vi "testing_waveforms.vi"() -> ()   [LabVIEW 2019, in "mmW_commands.lvlib"]
uses:
  mmW_commands.lvlib
  <vilib>/measure/maspectr.llb/FFT Power Spectrum and PSD for 1 Chan.vi
  <vilib>/measure/NI_MAPro.lvlib
  <vilib>/Analysis/NI_AALBase.lvlib
panel:
  out "theta":dbl[](graph)
  out "r":dbl[](graph)
  in  "cycles":dbl(slide)=400.0 scale=0.0..400.0
  out "Power Spectrum / PSD":cluster{"f0":dbl, "df":dbl, "magnitude":dbl[]}(graph)
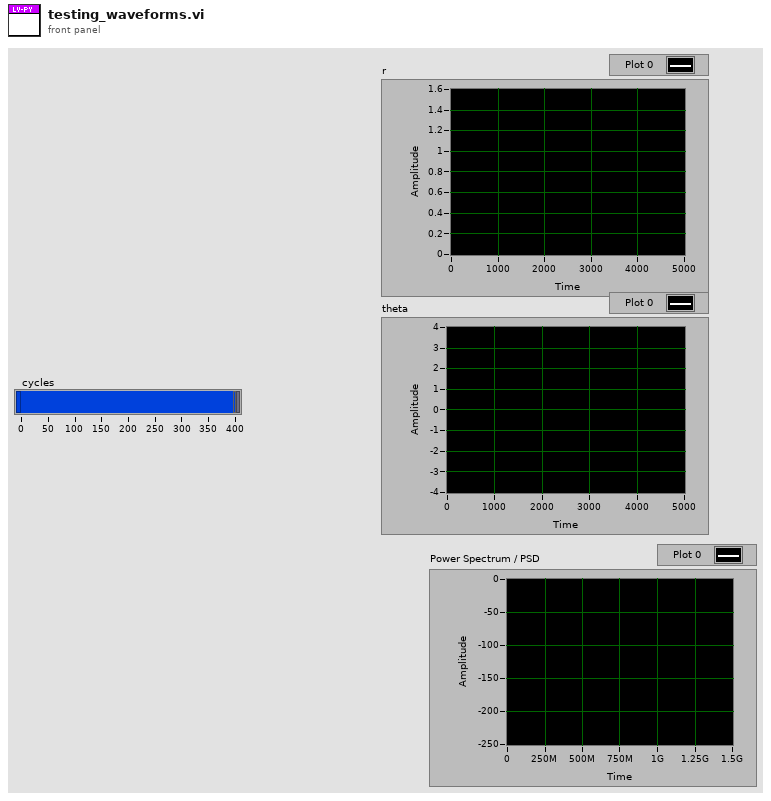
[diagram p1: front panel]
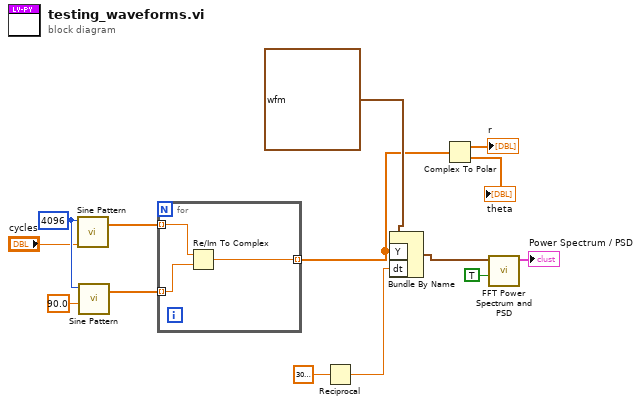
[diagram p0: block diagram]
diagram:
  w13 = 4096 ("samples")
  n1 = call <vilib>:"Sine Pattern.vi"("cycles"="cycles", "samples"=w13) -> ("Sinusoidal Pattern"=w12:dbl[])  [unwired: 2 in, 1 out]
  n2 = call <vilib>:"Sine Pattern.vi"("phase(degrees)"=90.0, "samples"=w13) -> ("Sinusoidal Pattern"=w11:dbl[])  [unwired: 2 in, 1 out]
  n3 = for {
    tunnel: w12 -> [w17] mode=indexing
    tunnel: w11 -> [w16] mode=indexing
    tunnel: [w15] -> w3 mode=indexing
    n4 = Re/Im To Complex(1:w16, 2:w17) -> (0:w15:cdb)
  }
  n5 = Reciprocal(x=3000000000.0) -> (1/x=w9:dbl)
  n6 = Bundle By Name(cluster=waveform(dbl) {"t0"=timestamp(0 s since 1904-01-01), "dt"=1.0, "Y"=[]} ("time signal"), "Y"=w3, "dt"=w9) -> (w7:waveform(dbl))
  n7 = Complex To Polar(r * e^(i*theta)=w3) -> (r=→"r":dbl[], theta=→"theta":dbl[])
  n8 = call-poly <vilib>:"FFT Power Spectrum and PSD.vi"("dB On (F)"=TRUE, "time signal"=w7) -> ("Power Spectrum / PSD"=→"Power Spectrum / PSD":cluster{"f0":dbl, "df":dbl, "magnitude":dbl[]})  [unwired: 6 in, 3 out]
